vi "Check HW Array Element Order.vi"(8 "error in (no error)":errorcluster, 9 "Compatible Hardware Types":string[](array[string]), 10 "Array of Hardware in":refnum<class "Hardware.lvclass">[](array[class]), 11 "Controller in":refnum<class "Controller.lvclass">) -> (0 "error out":errorcluster, 2 "Array of Hardware out":refnum<class "Hardware.lvclass">[](array[class]), 3 "Controller out":refnum<class "Controller.lvclass">)   [LabVIEW 2017, in "Controller Actor.lvlib" / "Controller.lvclass"]
uses:
  Controller.lvclass
  Hardware/Hardware.lvclass
  Hardware/Hardware.lvclass/Hardware.ctl
  <vilib>/Utility/LVClass/Get LV Class Path.vi
  <userlib>/_OpenG.lib/file/file.llb/Strip Path Extension__ogtk.vi
  <userlib>/_OpenG.lib/file/file.llb/Strip Path Extension - String__ogtk.vi
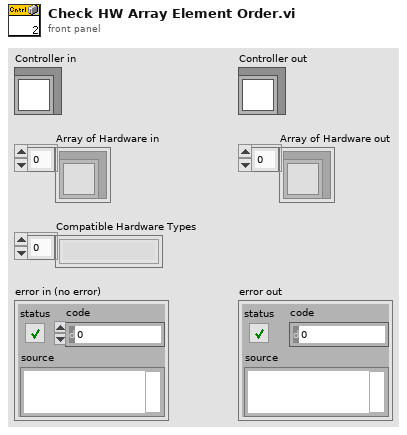
[diagram p1: front panel]
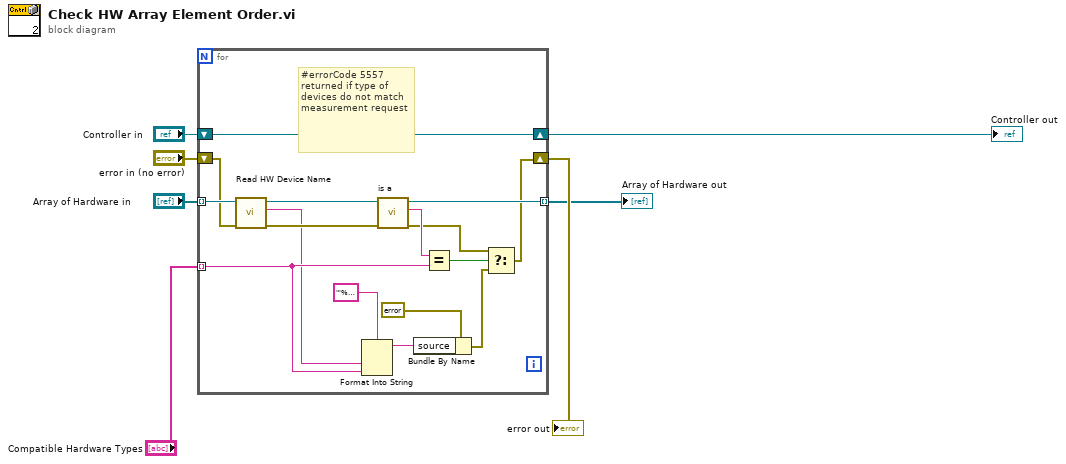
[diagram p0: block diagram]
diagram:
  n1 = for {
    shift-right: [w22] -> w1
    shift-left: "Controller in" -> [w22]
    shift-right: [w14] -> w6
    shift-left: "error in (no error)" -> [w10]
    tunnel: "Compatible Hardware Types" -> [w13] mode=indexing
    tunnel: [w23] -> w5 mode=indexing
    tunnel: "Array of Hardware in" -> [w12] mode=indexing
    # "#errorCode 5557 returned if type of devices do not match measurement request"
    n2 = call "Read HW Device Name.vi"("error in (no error)"=w10, "Analog in"=w12) -> ("error out"=w9:errorcluster, "Device Name"=w8:string, "Analog out"=w11:refnum<class "Hardware.lvclass">)  [unwired: 7 in]
    n3 = Format Into String(format string="'%s' is not compatible with measurement. A %s is required", w8, w13) -> (resulting string=w17:string)  [unwired: 2 in, 1 out]
    n4 = call-dynamic "is a.vi"("error in (no error)"=w9, "Hardware in"=w11) -> ("error out"=w15:errorcluster, "is a"=w21:string, "Hardware out"=w23:refnum<class "Hardware.lvclass">)  [unwired: 7 in]
    n5 = Bundle By Name(cluster=errorcluster {"status"=TRUE, "code"=5557, "source"=""} ("f"), "source"=w17) -> (w18:errorcluster)
    n6 = Equal?(x=w21, y=w13) -> (x = y?=w20:bool)
    n7 = Select(t=w15, s=w20, f=w18) -> (s? t:f=w14:errorcluster)
  }
  "error out" <- w6
  "Array of Hardware out" <- w5
  "Controller out" <- w1
